vi "NewScaleRawData_170907.vi"(4 "Vx,Vy,Vsum as signals or\ntrue X,Y,Z signal (1,default)":bool=TRUE, 5 "error in (no error)":errorcluster, 6 "All DAQ channels":T3, 7 "Scale Option":i32(ring)=2 items=["ScaleButDoNotCalculatePsi", "CalculatePsi, ButDoNotCompensate", "CompensationAllSignalsByCalcuatedPsi", "DoNotScale(ReadRawVoltageSignals)"], 8 "Params in":T8={"Manual Control"={"Rotation Control"={"Phase"=0.0, "A amp (0-120)"=75.0, "B amp (0-120)"=53.3, "mean freq  [MHz]\ndefault 39.99"=40.0, "freq difference [Hz]"=2.0, "Enable A"=TRUE, "Enable B"=TRUE}, "X piezo\n [nm]"=0.0, "Y peizo\n [nm]"=0.0, "-Z piezo\n [nm]"=5.012658227848101, "AOM0 \nPower"=0.2}, "Piezo Calibr"={"Px2Vx(AO)"=nan, "Py2Vy(AO)"=nan, "Pz2Vz(AO)"=nan, "Min Px"=nan, "Min Py"=nan, "Min Pz"=nan, "Max Px"=nan, "Max Py"=nan, "Max Pz"=nan, "Vx0 (V)"=nan, "Vy0 (V)"=nan, "Vz0 (V)"=nan}, "Instrument Calibr"={"Angular compensation coeffs"=[], "TetherCenter"={"TrapX_AO 0 [nm]"=nan, "TrapY_AO 0 [nm]"=nan, "TrapZ_AO 0 [nm]"=nan}, "XYZsignal baseline"={"Xsignal0"=nan, "Ysignal0"=nan, "Zsignal0"=nan, "Zsig slope"=nan, "Z bead0"=nan}, "S and P to Vs0"={"Vs0/P"=1.0, "Vs0/S"=1.0}, "Psi"=0.0, "ePS:eRL drift correlation"={"Interc P"=nan, "Slope P"=nan, "Interc S"=nan, "Slope S"=nan}, "Current piezo volt AO"={"Vpx_AO [V]"=nan, "Vpy_AO [V]"=nan, "Vpz_AO [V]"=nan}}, "Cylinder Calibr"={"ZStiff"=nan, "Zsens"=nan, "AngStiff"=nan, "XStiff"=nan, "Xsens"=nan, "MaxEllip"=nan, "YStiff"=nan, "Ysens"=nan, "FocalShift"=nan, "Sfz"=nan, "1/Sz"=nan, "Stau"=nan, "Sfx"=nan, "1/Sx"=nan, "1/Sang"=nan, "Sfy"=nan, "1/Sy"=nan, "1/focal"=nan}, "DAQParams"={"Buffer size"=nan, "Scanning rate"=nan, "Average"=nan, "Sampling rate"=nan, "set dt"=nan}, "DAQ channel offsets"={"A0 [V]"=0.0, "D0 [V]"=0.0, "P0  [V]"=0.0, "S0 [V]"=0.0, "L0 [V]"=0.0, "R0 [V]"=0.0, "Vpx0 [V]"=0.0, "Vpy0 [V]"=0.0, "Vpz0 [V]"=0.0, "Vsum0 [V]"=0.0, "Vpx_AO0 [V]"=0.0, "Vpy_AO0 [V]"=0.0, "Vpz_AO0 [V]"=0.0}, "Z bead polynomial coeffs"=[nan, nan, nan, nan], "Skip button ref"=refnum, "z bead lookup table"={"z signal"=[], "z bead"=[]}, "SP->power Matrix"=[], "Ms2p"=[], "Mp2s"=[], "Polynomial coeff V_px,y,z 2 position (nm)"=[], "task in"=""} {"Instrument Calibr"."Psi" format="%#_2f"; "Manual Control"."Y peizo\n [nm]" scale=0.0..7000.0; "Manual Control"."AOM0 \nPower" scale=0.0..1.0; "Manual Control"."X piezo\n [nm]" scale=0.0..7000.0; "Manual Control"."Rotation Control"."freq difference [Hz]" step=0.5; "Manual Control"."Rotation Control"."mean freq  [MHz]\ndefault 39.99" min=0.0 step=0.01; "Manual Control"."Rotation Control"."B amp (0-120)" min=0.0 max=120.0 step=0.1; "Manual Control"."Rotation Control"."A amp (0-120)" min=0.0 max=120.0 step=0.1; "Manual Control"."Rotation Control"."Phase" scale=0.0..360.0; "Manual Control"."-Z piezo\n [nm]" scale=1000.0..7000.0}) -> (0 "error out":errorcluster, 1 "Scaled data":T7, 2 "All DAQ channels out":T3, 3 "Params out":T8={"Manual Control"={"Rotation Control"={"Phase"=0.0, "A amp (0-120)"=75.0, "B amp (0-120)"=53.3, "mean freq  [MHz]\ndefault 39.99"=40.0, "freq difference [Hz]"=2.0, "Enable A"=TRUE, "Enable B"=TRUE}, "X piezo\n [nm]"=0.0, "Y peizo\n [nm]"=0.0, "-Z piezo\n [nm]"=5.012658227848101, "AOM0 \nPower"=0.2}, "Piezo Calibr"={"Px2Vx(AO)"=nan, "Py2Vy(AO)"=nan, "Pz2Vz(AO)"=nan, "Min Px"=nan, "Min Py"=nan, "Min Pz"=nan, "Max Px"=nan, "Max Py"=nan, "Max Pz"=nan, "Vx0 (V)"=nan, "Vy0 (V)"=nan, "Vz0 (V)"=nan}, "Instrument Calibr"={"Angular compensation coeffs"=[], "TetherCenter"={"TrapX_AO 0 [nm]"=nan, "TrapY_AO 0 [nm]"=nan, "TrapZ_AO 0 [nm]"=nan}, "XYZsignal baseline"={"Xsignal0"=nan, "Ysignal0"=nan, "Zsignal0"=nan, "Zsig slope"=nan, "Z bead0"=nan}, "S and P to Vs0"={"Vs0/P"=1.0, "Vs0/S"=1.0}, "Psi"=0.0, "ePS:eRL drift correlation"={"Interc P"=nan, "Slope P"=nan, "Interc S"=nan, "Slope S"=nan}, "Current piezo volt AO"={"Vpx_AO [V]"=nan, "Vpy_AO [V]"=nan, "Vpz_AO [V]"=nan}}, "Cylinder Calibr"={"ZStiff"=nan, "Zsens"=nan, "AngStiff"=nan, "XStiff"=nan, "Xsens"=nan, "MaxEllip"=nan, "YStiff"=nan, "Ysens"=nan, "FocalShift"=nan, "Sfz"=nan, "1/Sz"=nan, "Stau"=nan, "Sfx"=nan, "1/Sx"=nan, "1/Sang"=nan, "Sfy"=nan, "1/Sy"=nan, "1/focal"=nan}, "DAQParams"={"Buffer size"=nan, "Scanning rate"=nan, "Average"=nan, "Sampling rate"=nan, "set dt"=nan}, "DAQ channel offsets"={"A0 [V]"=0.0, "D0 [V]"=0.0, "P0  [V]"=0.0, "S0 [V]"=0.0, "L0 [V]"=0.0, "R0 [V]"=0.0, "Vpx0 [V]"=0.0, "Vpy0 [V]"=0.0, "Vpz0 [V]"=0.0, "Vsum0 [V]"=0.0, "Vpx_AO0 [V]"=0.0, "Vpy_AO0 [V]"=0.0, "Vpz_AO0 [V]"=0.0}, "Z bead polynomial coeffs"=[nan, nan, nan, nan], "Skip button ref"=refnum, "z bead lookup table"={"z signal"=[], "z bead"=[]}, "SP->power Matrix"=[], "Ms2p"=[], "Mp2s"=[], "Polynomial coeff V_px,y,z 2 position (nm)"=[], "task in"=""} {"Instrument Calibr"."Psi" format="%#_2f"; "Manual Control"."Y peizo\n [nm]" scale=0.0..7000.0; "Manual Control"."AOM0 \nPower" scale=0.0..1.0; "Manual Control"."X piezo\n [nm]" scale=0.0..7000.0; "Manual Control"."Rotation Control"."freq difference [Hz]" step=0.5; "Manual Control"."Rotation Control"."mean freq  [MHz]\ndefault 39.99" min=0.0 step=0.01; "Manual Control"."Rotation Control"."B amp (0-120)" min=0.0 max=120.0 step=0.1; "Manual Control"."Rotation Control"."A amp (0-120)" min=0.0 max=120.0 step=0.1; "Manual Control"."Rotation Control"."Phase" scale=0.0..360.0; "Manual Control"."-Z piezo\n [nm]" scale=1000.0..7000.0})   [LabVIEW 2017, in "SignalConverson.lvlib"]
uses:
  SignalConverson.lvlib
  Initialization/New Param_170907.ctl
  Initialization/ManualCtrl.ctl
  Initialization/CylinderCalibrNew.ctl
  DAQChannelOffsets.ctl
  <vilib>/Analysis/Matrix/Datatypes/RealMatrix.ctl
  DAQChannelRawData.ctl
  ScaledData.ctl
  Measrured TrapXYZ.ctl
  Data Before Angle Compensation.ctl
  Angle compensated data.ctl
  XYZ Signals.ctl
  Set TrapXYZ.ctl
  <vilib>/Analysis/baseanly.llb/A x Vector.vi
  <vilib>/Analysis/polynomials.llb/Scalar Polynomial Evaluation (DBL).vi
  <vilib>/Analysis/NI_AALBase.lvlib
  <vilib>/Analysis/NI_AALPro.lvlib
  Initialization/Initialization.lvlib
  <vilib>/Analysis/Matrix/NI_Matrix.lvlib
panel:
  out "Data before TCT":T1
  out "set TrapXYZ":T2
  out "Measured Piezo Position":T4
  out "X,Y,Z signal":T5
  out "Data after TCT":T6
  out "Data Before TCT":T1
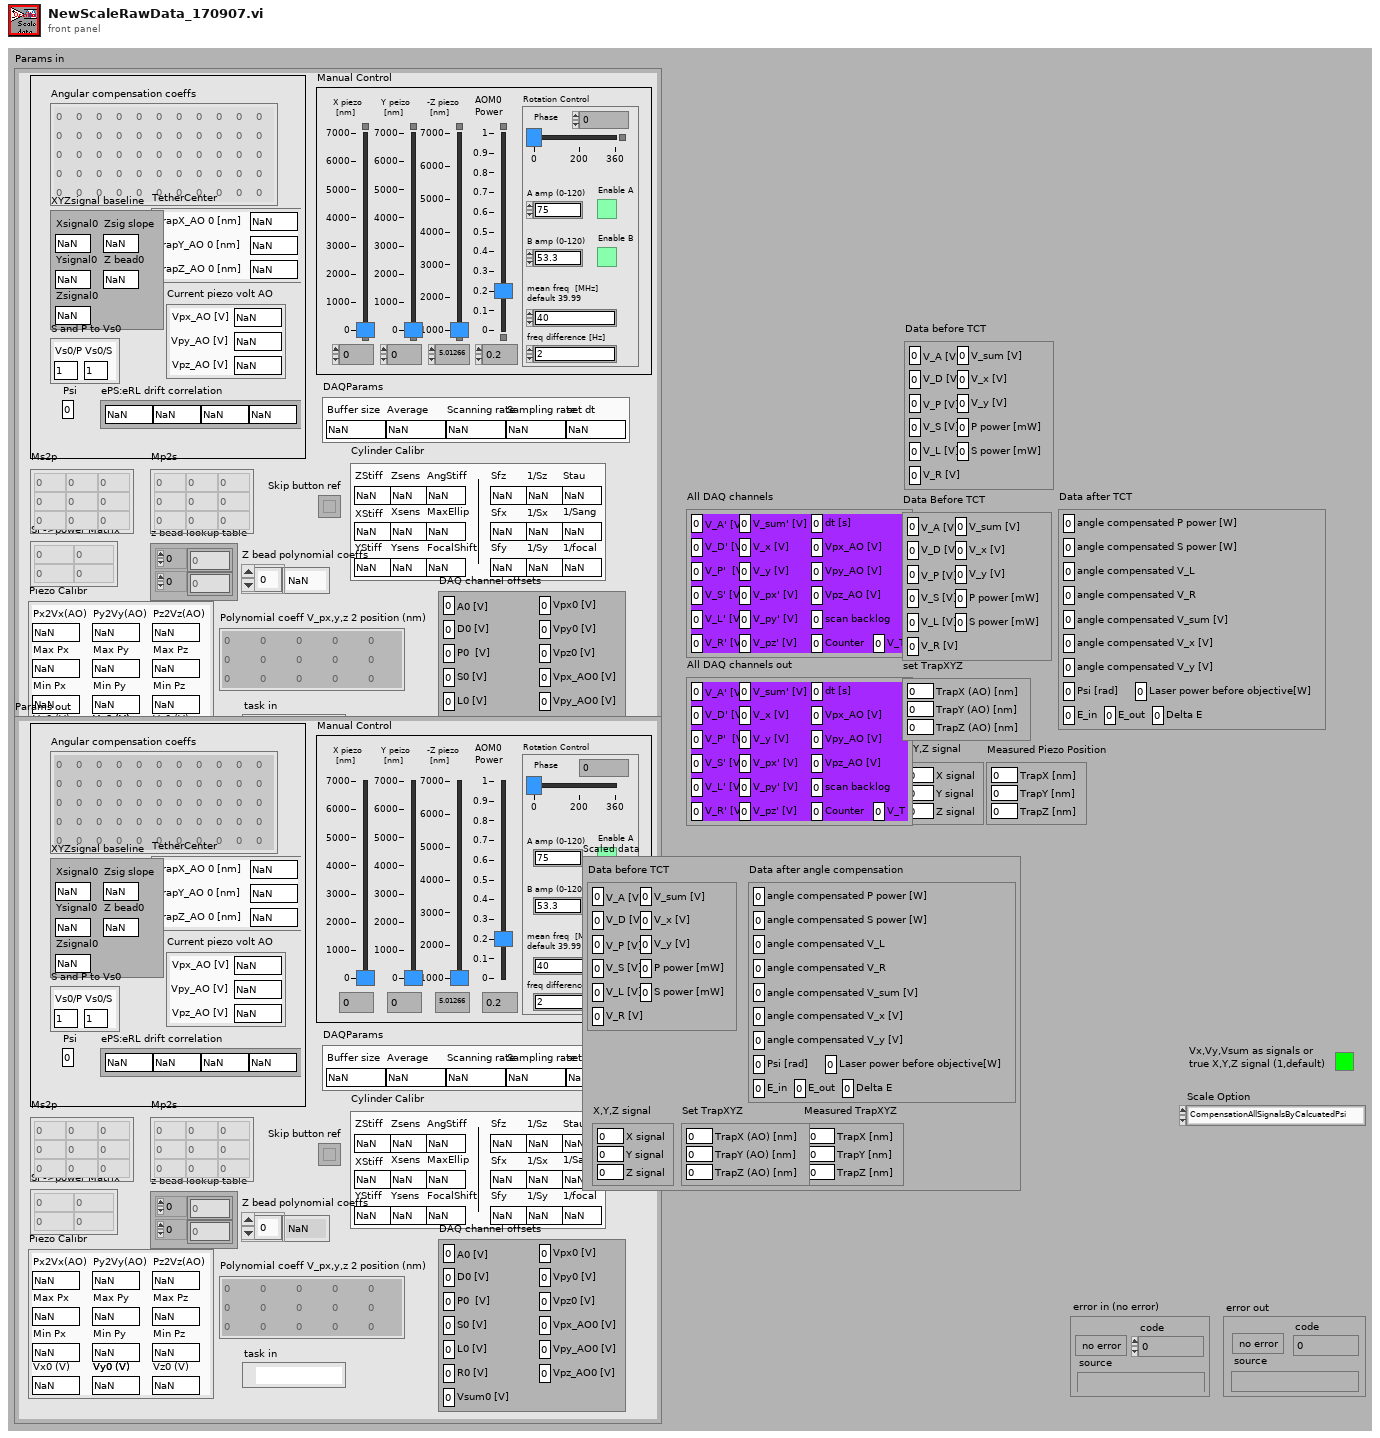
[diagram p1: front panel]
types:
  T1 = typedef "SignalConverson.lvlib/Data Before Angle Compensation.ctl" = cluster{"V_A [V]":dbl, "V_D [V]":dbl, "V_P [V]":dbl, "V_S [V]":dbl, "V_L [V]":dbl, "V_R [V]":dbl, "V_sum [V]":dbl, "V_x [V]":dbl, "V_y [V]":dbl, "P power [mW]":dbl, "S power [mW]":dbl}
  T2 = typedef "SignalConverson.lvlib/Set TrapXYZ.ctl" = cluster{"TrapX (AO) [nm]":dbl, "TrapY (AO) [nm]":dbl, "TrapZ (AO) [nm]":dbl}
  T3 = typedef "SignalConverson.lvlib/DAQChannelRawData.ctl" = cluster{"V_A' [V]":dbl, "V_D' [V]":dbl, "V_P'  [V]":dbl, "V_S' [V]":dbl, "V_L' [V]":dbl, "V_R' [V]":dbl, "V_sum' [V]":dbl, "V_x [V]":dbl, "V_y [V]":dbl, "V_px' [V]":dbl, "V_py' [V]":dbl, "V_pz' [V]":dbl, "dt [s]":dbl, "Vpx_AO [V]":dbl, "Vpy_AO [V]":dbl, "Vpz_AO [V]":dbl, "scan backlog":u32, "Counter":u32, "V_T":dbl}
  T4 = typedef "SignalConverson.lvlib/Measrured TrapXYZ.ctl" = cluster{"TrapX [nm]":dbl, "TrapY [nm]":dbl, "TrapZ [nm]":dbl}
  T5 = typedef "SignalConverson.lvlib/XYZ Signals.ctl" = cluster{"X signal":dbl, "Y signal":dbl, "Z signal":dbl}
  T6 = typedef "SignalConverson.lvlib/Angle compensated data.ctl" = cluster{"angle compensated P power [W]":dbl, "angle compensated S power [W]":dbl, "angle compensated V_L":dbl, "angle compensated V_R":dbl, "angle compensated V_sum [V]":dbl, "angle compensated V_x [V]":dbl, "angle compensated V_y [V]":dbl, "Psi [rad]":dbl, "Laser power before objective[W]":dbl, "E_in":dbl, "E_out":dbl, "Delta E":dbl}
  T7 = typedef "SignalConverson.lvlib/ScaledData.ctl" = cluster{"Measured TrapXYZ":T4, "Data before TCT":T1, "Data after angle compensation":T6, "X,Y,Z signal":T5, "Set TrapXYZ":T2}
  T8 = typedef "Initialization.lvlib/New Param_170907.ctl" = cluster{"Manual Control":T9, "Piezo Calibr":cluster{"Px2Vx(AO)":dbl, "Py2Vy(AO)":dbl, "Pz2Vz(AO)":dbl, "Min Px":dbl, "Min Py":dbl, "Min Pz":dbl, "Max Px":dbl, "Max Py":dbl, "Max Pz":dbl, "Vx0 (V)":dbl, "Vy0 (V)":dbl, "Vz0 (V)":dbl}, "Instrument Calibr":cluster{"Angular compensation coeffs":dbl[][], "TetherCenter":cluster{"TrapX_AO 0 [nm]":dbl, "TrapY_AO 0 [nm]":dbl, "TrapZ_AO 0 [nm]":dbl}, "XYZsignal baseline":cluster{"Xsignal0":dbl, "Ysignal0":dbl, "Zsignal0":dbl, "Zsig slope":dbl, "Z bead0":dbl}, "S and P to Vs0":cluster{"Vs0/P":dbl, "Vs0/S":dbl}, "Psi":dbl, "ePS:eRL drift correlation":cluster{"Interc P":dbl, "Slope P":dbl, "Interc S":dbl, "Slope S":dbl}, "Current piezo volt AO":cluster{"Vpx_AO [V]":dbl, "Vpy_AO [V]":dbl, "Vpz_AO [V]":dbl}}, "Cylinder Calibr":T10, "DAQParams":cluster{"Buffer size":dbl, "Scanning rate":dbl, "Average":dbl, "Sampling rate":dbl, "set dt":dbl}, "DAQ channel offsets":T11, "Z bead polynomial coeffs":dbl[], "Skip button ref":refnum<vi>, "z bead lookup table":cluster{"z signal":dbl[], "z bead":dbl[]}, "SP->power Matrix":T12, "Ms2p":T12, "Mp2s":T12, "Polynomial coeff V_px,y,z 2 position (nm)":dbl[][], "task in":refnum<k21>}
  T9 = typedef "Initialization.lvlib/ManualCtrl.ctl" = cluster{"Rotation Control":cluster{"Phase":dbl, "A amp (0-120)":dbl, "B amp (0-120)":dbl, "mean freq  [MHz]\ndefault 39.99":dbl, "freq difference [Hz]":dbl, "Enable A":bool, "Enable B":bool}, "X piezo\n [nm]":dbl, "Y peizo\n [nm]":dbl, "-Z piezo\n [nm]":dbl, "AOM0 \nPower":dbl}
  T10 = typedef "Initialization.lvlib/CylinderCalibrNew.ctl" = cluster{"ZStiff":dbl, "Zsens":dbl, "AngStiff":dbl, "XStiff":dbl, "Xsens":dbl, "MaxEllip":dbl, "YStiff":dbl, "Ysens":dbl, "FocalShift":dbl, "Sfz":dbl, "1/Sz":dbl, "Stau":dbl, "Sfx":dbl, "1/Sx":dbl, "1/Sang":dbl, "Sfy":dbl, "1/Sy":dbl, "1/focal":dbl}
  T11 = typedef "SignalConverson.lvlib/DAQChannelOffsets.ctl" = cluster{"A0 [V]":dbl, "D0 [V]":dbl, "P0  [V]":dbl, "S0 [V]":dbl, "L0 [V]":dbl, "R0 [V]":dbl, "Vpx0 [V]":dbl, "Vpy0 [V]":dbl, "Vpz0 [V]":dbl, "Vsum0 [V]":dbl, "Vpx_AO0 [V]":dbl, "Vpy_AO0 [V]":dbl, "Vpz_AO0 [V]":dbl}
  T12 = typedef "NI_Matrix.lvlib/RealMatrix.ctl" = dbl[][]
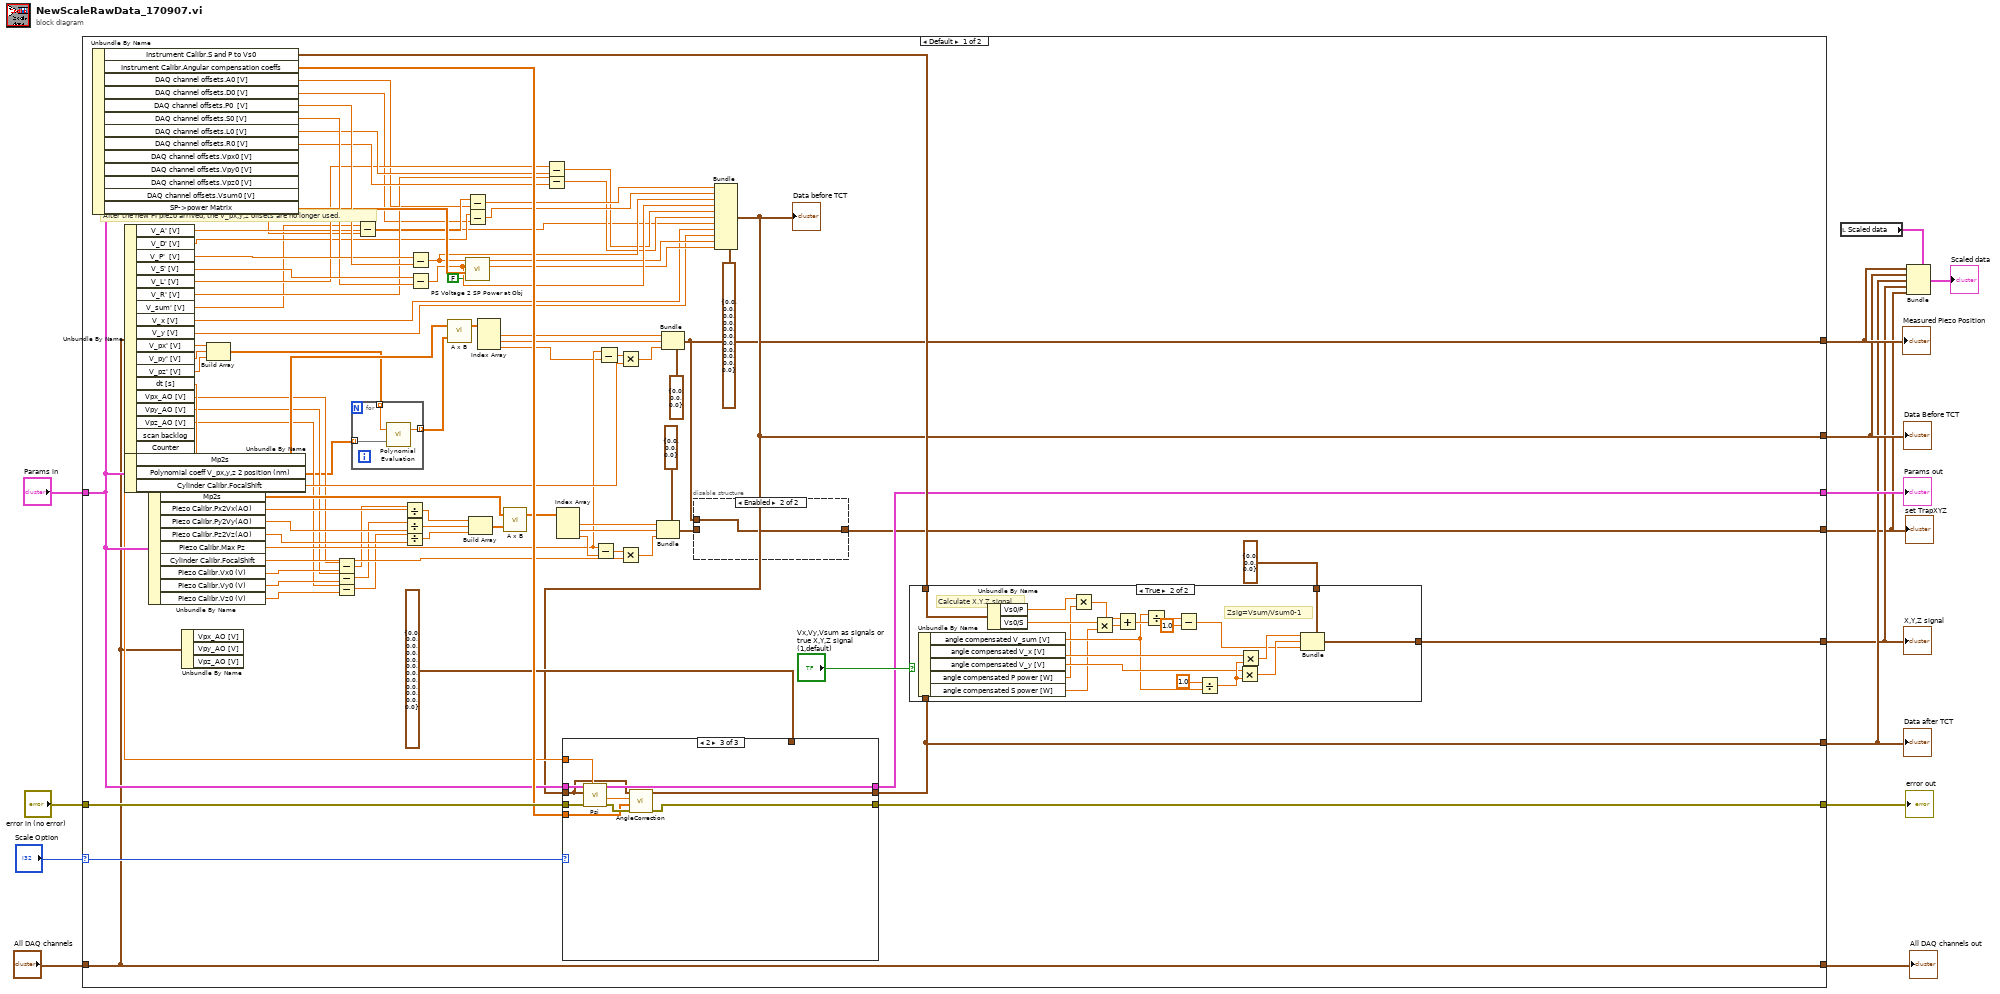
[diagram p0: block diagram]
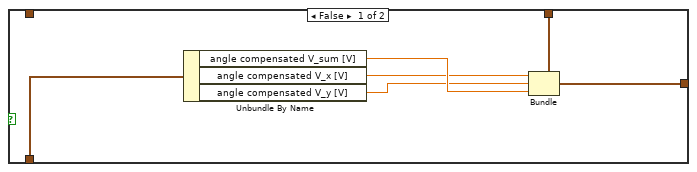
[diagram p3: hidden frame]
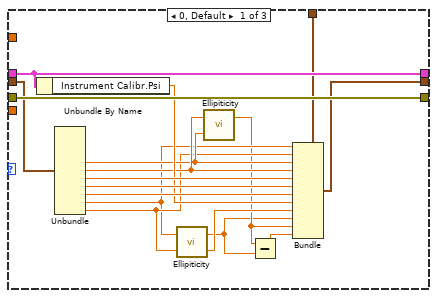
[diagram p4: hidden frame]
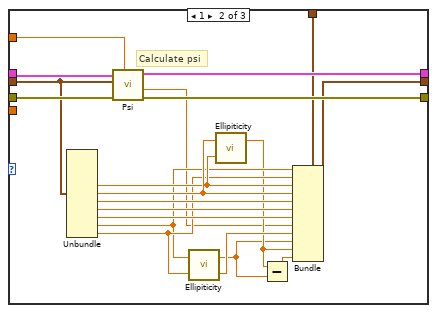
[diagram p5: hidden frame]
diagram:
  n1 = case shown="Default" "Scale Option" {
    selector: "Scale Option" -> [w98 _]
    tunnel: "All DAQ channels" -> [w51 w181]
    tunnel: "Params in" -> [w86 w182]
    tunnel: "error in (no error)" -> [w101 w183]
    tunnel: [w99 w183] -> w2
    tunnel: [w95 w182] -> w13
    tunnel: [w56 _] -> w4
    tunnel: [w55 _] -> w5
    tunnel: [w42 _] -> w6
    tunnel: [w16 _] -> w7
    tunnel: [w51 w181] -> w9
    tunnel: [w17 _] -> w3
    frame Default {
      # "After the new PI piezo arrived, the V_px,y,z offsets are no longer used."
      n2 = Unbundle By Name(w86) -> ("Instrument Calibr.S and P to Vs0"=w97:cluster{"Vs0/P":dbl, "Vs0/S":dbl}, "Instrument Calibr.Angular compensation coeffs"=w100:dbl[][], "DAQ channel offsets.A0 [V]"=w71:dbl, "DAQ channel offsets.D0 [V]"=w70:dbl, "DAQ channel offsets.P0  [V]"=w94:dbl, "DAQ channel offsets.S0 [V]"=w91:dbl, "DAQ channel offsets.L0 [V]"=w84:dbl, "DAQ channel offsets.R0 [V]"=w85:dbl, "DAQ channel offsets.Vsum0 [V]"=w40:dbl, "SP->power Matrix"=w90:T12)  [unwired: 3 out]
      n3 = Unbundle By Name(w86) -> ("Mp2s"=w87:T12, "Polynomial coeff V_px,y,z 2 position (nm)"=w24:dbl[][], "Cylinder Calibr.FocalShift"=w88:dbl)
      n4 = Unbundle By Name(w51) -> ("V_A' [V]"=w73:dbl, "V_D' [V]"=w72:dbl, "V_P'  [V]"=w93:dbl, "V_S' [V]"=w92:dbl, "V_L' [V]"=w83:dbl, "V_R' [V]"=w82:dbl, "V_sum' [V]"=w39:dbl, "V_x [V]"=w61:dbl, "V_y [V]"=w60:dbl, "V_px' [V]"=w21:dbl, "V_py' [V]"=w20:dbl, "V_pz' [V]"=w19:dbl, "dt [s]"=w59:dbl, "Vpx_AO [V]"=w30:dbl, "Vpy_AO [V]"=w29:dbl, "Vpz_AO [V]"=w28:dbl)  [unwired: 2 out]
      n5 = Unbundle By Name(w86) -> ("Mp2s"=w75:T12, "Piezo Calibr.Px2Vx(AO)"=w81:dbl, "Piezo Calibr.Py2Vy(AO)"=w80:dbl, "Piezo Calibr.Pz2Vz(AO)"=w79:dbl, "Piezo Calibr.Max Pz"=w37:dbl, "Cylinder Calibr.FocalShift"=w47:dbl, "Piezo Calibr.Vx0 (V)"=w33:dbl, "Piezo Calibr.Vy0 (V)"=w32:dbl, "Piezo Calibr.Vz0 (V)"=w31:dbl)
      n6 = Unbundle By Name(w51) -> ()  [unwired: 3 out]
      n7 = Build Array(w21, w20, w19) -> (w23:dbl[])
      n8 = Subtract(x=w30, y=w33) -> (x-y=w27:dbl)
      n9 = Subtract(x=w29, y=w32) -> (x-y=w26:dbl)
      n10 = Subtract(x=w28, y=w31) -> (x-y=w25:dbl)
      n11 = for {
        tunnel: w24 -> [w105] mode=indexing
        tunnel: w23 -> [w106] mode=indexing
        tunnel: [w104] -> w22 mode=indexing
        n12 = call-poly <vilib>:"Polynomial Evaluation.vi"("P(x)"=w105, "a"=w106) -> ("P(a)"=w104:dbl)  [unwired: 1 out]
      }
      n13 = Subtract(x=w39, y=w40) -> (x-y=w38:dbl)
      n14 = Divide(x=w27, y=w81) -> (x/y=w77:dbl)
      n15 = Divide(x=w26, y=w80) -> (x/y=w78:dbl)
      n16 = Divide(x=w25, y=w79) -> (x/y=w50:dbl)
      n17 = Subtract(x=w93, y=w94) -> (x-y=w67:dbl)
      n18 = Subtract(x=w92, y=w91) -> (x-y=w66:dbl)
      n19 = call-poly <vilib>:"A x B.vi"("Vector"=w22, "A"=w87) -> ("A x Vector"=w89:dbl[])  [unwired: 1 out]
      n20 = Subtract(x=w73, y=w71) -> (x-y=w69:dbl)
      n21 = Subtract(x=w72, y=w70) -> (x-y=w68:dbl)
      n22 = call "PS Voltage 2 SP Power at Obj.vi"("Switch"=FALSE, "SP -> Power Matrix"=w90, "Volts S"=w66, "Volts P"=w67) -> ("Power S"=w62:dbl, "Power P"=w63:dbl)  [unwired: 2 in]
      n23 = Build Array(w77, w78, w50) -> (w76:dbl[])
      n24 = Index Array(array=w89) -> (element #1=w53:dbl, element #2=w52:dbl, element #3=w36:dbl)  [unwired: 3 in]
      n25 = call-poly <vilib>:"A x B.vi"("Vector"=w76, "A"=w75) -> ("A x Vector"=w74:dbl[])  [unwired: 1 out]
      n26 = Subtract(x=w83, y=w84) -> (x-y=w65:dbl)
      n27 = Subtract(x=w82, y=w85) -> (x-y=w64:dbl)
      n28 = Index Array(array=w74) -> (element #1=w46:dbl, element #2=w45:dbl, element #3=w49:dbl)  [unwired: 3 in]
      n29 = Subtract(x=w37, y=w49) -> (x-y=w48:dbl)
      n30 = Subtract(x=w37, y=w36) -> (x-y=w35:dbl)
      n31 = Multiply(x=w48, y=w47) -> (x*y=w44:dbl)
      n32 = Multiply(x=w35, y=w88) -> (x*y=w34:dbl)
      n33 = Bundle(cluster=T2 {"TrapX (AO) [nm]"=0.0, "TrapY (AO) [nm]"=0.0, "TrapZ (AO) [nm]"=0.0} ("set TrapXYZ"), "TrapX (AO) [nm]"=w46, "TrapY (AO) [nm]"=w45, "TrapZ (AO) [nm]"=w44) -> (w18:T2)
      n34 = Bundle(cluster=T4 {"TrapX [nm]"=0.0, "TrapY [nm]"=0.0, "TrapZ [nm]"=0.0} ("Measured Piezo Position"), "TrapX [nm]"=w53, "TrapY [nm]"=w52, "TrapZ [nm]"=w34) -> (w16:T4)
      n35 = disable-structure shown="Enabled" {
        disable-tunnel: w18 -> [w102 _]
        disable-tunnel: [w102 w103] -> w17
        disable-tunnel: w16 -> [_ w103]
        frame Disabled {
          # "There's no set piezo voltage"
        }
        frame Enabled {
        }
      }
      n36 = Bundle(cluster=T1 {"V_A [V]"=0.0, "V_D [V]"=0.0, "V_P [V]"=0.0, "V_S [V]"=0.0, "V_L [V]"=0.0, "V_R [V]"=0.0, "V_sum [V]"=0.0, "V_x [V]"=0.0, "V_y [V]"=0.0, "P power [mW]"=0.0, "S power [mW]"=0.0} ("Data before TCT"), "V_A [V]"=w69, "V_D [V]"=w68, "V_P [V]"=w67, "V_S [V]"=w66, "V_L [V]"=w65, "V_R [V]"=w64, "V_sum [V]"=w38, "V_x [V]"=w61, "V_y [V]"=w60, "P power [mW]"=w63, "S power [mW]"=w62) -> (w42:T1)
      "Data before TCT" <- w42
      n37 = case shown="2" w98 {
        tunnel: w101 -> [w150 w169 w179]
        tunnel: [w142 w152 w172] -> w55
        tunnel: [w150 w170 w178] -> w99
        tunnel: w100 -> [_ _ w177]
        tunnel: w86 -> [w149 w168 w176]
        tunnel: [w149 w167 w175] -> w95
        tunnel: w42 -> [w148 w154 w171]
        tunnel: w59 -> [_ w166 w173]
        tunnel: T6 {"angle compensated P power [W]"=0.0, "angle compensated S power [W]"=0.0, "angle compensated V_L"=0.0, "angle compensated V_R"=0.0, "angle compensated V_sum [V]"=0.0, "angle compensated V_x [V]"=0.0, "angle compensated V_y [V]"=0.0, "Psi [rad]"=0.0, "Laser power before objective[W]"=0.0, "E_in"=0.0, "E_out"=0.0, "Delta E"=0.0} ("Data after TCT") -> [w147 w153 _]
        frame 0, Default {
          n38 = Unbundle By Name(w149) -> ("Instrument Calibr.Psi"=w143:dbl)
          n39 = Unbundle(w148) -> ("V_L [V]"=w140:dbl, "V_R [V]"=w141:dbl, "V_sum [V]"=w146:dbl, "V_x [V]"=w145:dbl, "V_y [V]"=w144:dbl, "P power [mW]"=w138:dbl, "S power [mW]"=w139:dbl)  [unwired: 4 out]
          n40 = call "Ellipiticity.vi"("S"=w139, "P"=w138) -> ("P+S"=w137:dbl, "(P-S)/(P+S)"=w135:dbl)
          n41 = call "Ellipiticity.vi"("S"=w140, "P"=w141) -> ("(P-S)/(P+S)"=w136:dbl)  [unwired: 1 out]
          n42 = Subtract(x=w136, y=w135) -> (x-y=w134:dbl)
          n43 = Bundle(cluster=w147, "angle compensated P power [W]"=w138, "angle compensated S power [W]"=w139, "angle compensated V_L"=w140, "angle compensated V_R"=w141, "angle compensated V_sum [V]"=w146, "angle compensated V_x [V]"=w145, "angle compensated V_y [V]"=w144, "Psi [rad]"=w143, "Laser power before objective[W]"=w137, "E_in"=w135, "E_out"=w136, "Delta E"=w134) -> (w142:T6)
        }
        frame 1 {
          # "Calculate psi"
          n44 = Unbundle(w154) -> ("V_L [V]"=w161:dbl, "V_R [V]"=w162:dbl, "V_sum [V]"=w165:dbl, "V_x [V]"=w164:dbl, "V_y [V]"=w163:dbl, "P power [mW]"=w159:dbl, "S power [mW]"=w160:dbl)  [unwired: 4 out]
          n45 = call "Psi.vi"("dt [s]"=w166, "error in (no error)"=w169, "Data before TCT"=w154, "Params in"=w168) -> ("error out"=w170:errorcluster, "Psi"=w151:dbl, "Params out"=w167:T8)  [unwired: 2 in]
          n46 = call "Ellipiticity.vi"("S"=w160, "P"=w159) -> ("P+S"=w158:dbl, "(P-S)/(P+S)"=w156:dbl)
          n47 = call "Ellipiticity.vi"("S"=w161, "P"=w162) -> ("(P-S)/(P+S)"=w157:dbl)  [unwired: 1 out]
          n48 = Subtract(x=w157, y=w156) -> (x-y=w155:dbl)
          n49 = Bundle(cluster=w153, "angle compensated P power [W]"=w159, "angle compensated S power [W]"=w160, "angle compensated V_L"=w161, "angle compensated V_R"=w162, "angle compensated V_sum [V]"=w165, "angle compensated V_x [V]"=w164, "angle compensated V_y [V]"=w163, "Psi [rad]"=w151, "Laser power before objective[W]"=w158, "E_in"=w156, "E_out"=w157, "Delta E"=w155) -> (w152:T6)
        }
        frame 2 {
          n50 = call "Psi.vi"("dt [s]"=w173, "error in (no error)"=w179, "Data before TCT"=w171, "Params in"=w176) -> ("error out"=w180:errorcluster, "Psi"=w174:dbl, "Params out"=w175:T8)  [unwired: 2 in]
          n51 = call "AngleCorrection.vi"("error in (no error)"=w180, "TQGT"=w177, "Psi"=w174, "Data Before TCT"=w171) -> ("error out"=w178:errorcluster, "Data after TCT"=w172:T6)  [unwired: 2 in]
        }
      }
      n52 = case shown="True" "Vx,Vy,Vsum as signals or\ntrue X,Y,Z signal (1,default)" {
        tunnel: w97 -> [_ w126]
        tunnel: [w111 w114] -> w56
        tunnel: w55 -> [w110 w123]
        tunnel: T5 {"X signal"=0.0, "Y signal"=0.0, "Z signal"=0.0} ("X,Y,Z signal") -> [w112 w113]
        frame False {
          n53 = Unbundle By Name(w110) -> ("angle compensated V_sum [V]"=w109:dbl, "angle compensated V_x [V]"=w108:dbl, "angle compensated V_y [V]"=w107:dbl)
          n54 = Bundle(cluster=w112, "X signal"=w108, "Y signal"=w107, "Z signal"=w109) -> (w111:T5)
        }
        frame True {
          # "Zsig=Vsum/Vsum0-1"
          # "Calculate X.Y.Z signal"
          n55 = Unbundle By Name(w123) -> ("angle compensated V_sum [V]"=w120:dbl, "angle compensated V_x [V]"=w122:dbl, "angle compensated V_y [V]"=w121:dbl, "angle compensated P power [W]"=w119:dbl, "angle compensated S power [W]"=w118:dbl)
          n56 = Unbundle By Name(w126) -> ("Vs0/P"=w129:dbl, "Vs0/S"=w130:dbl)
          n57 = Multiply(x=w129, y=w119) -> (x*y=w132:dbl)
          n58 = Multiply(x=w130, y=w118) -> (x*y=w131:dbl)
          n59 = Add(x=w132, y=w131) -> (x+y=w133:dbl)
          n60 = Divide(x=w120, y=w133) -> (x/y=w125:dbl)
          n61 = Subtract(x=w125, y=1.0 ("x")) -> (x-y=w115:dbl)
          n62 = Divide(x=1.0, y=w120) -> (x/y=w128:dbl)
          n63 = Multiply(x=w121, y=w128) -> (x*y=w116:dbl)
          n64 = Multiply(x=w122, y=w128) -> (x*y=w117:dbl)
          n65 = Bundle(cluster=w113, "X signal"=w117, "Y signal"=w116, "Z signal"=w115) -> (w114:T5)
        }
      }
    }
    frame 3 {
    }
  }
  "Params out" <- w13
  "X,Y,Z signal" <- w4
  "Data after TCT" <- w5
  "Data Before TCT" <- w6
  "Measured Piezo Position" <- w7
  "All DAQ channels out" <- w9
  "set TrapXYZ" <- w3
  "error out" <- w2
  n66 = local read "Scaled data"() -> (w8:T7)
  n67 = Bundle(cluster=w8, "Measured TrapXYZ"=w7, "Data before TCT"=w6, "Data after angle compensation"=w5, "X,Y,Z signal"=w4, "Set TrapXYZ"=w3) -> (→"Scaled data":T7)
